vi "Wrapper_Get Image Frame.vi"(7 "Image Ref in":T4, 8 "error in (no error)":errorcluster, 9 "frameindex in":i32, 10 "LIMPICTURE in":T2, 11 "hFile in":T3) -> (0 "error out":errorcluster, 1 "LIMLOCALMETADATA":T1 {"dTimeMSec" format="%.2f"}, 2 "LIMPICTURE out":T2, 3 "hFile out":T3, 5 "Image Ref out":T4)   [LabVIEW 2014, in "ND2_Reader_32.lvlib"]
uses:
  ND2_Reader_32.lvlib
  <vilib>/vision/Image Controls.llb/IMAQ Image.ctl
  controls/numeric_LIMFILEHANDLE.ctl
  controls/cluster_LIMPICTURE.ctl
  controls/cluster_LIMLOCALMETADATA.ctl
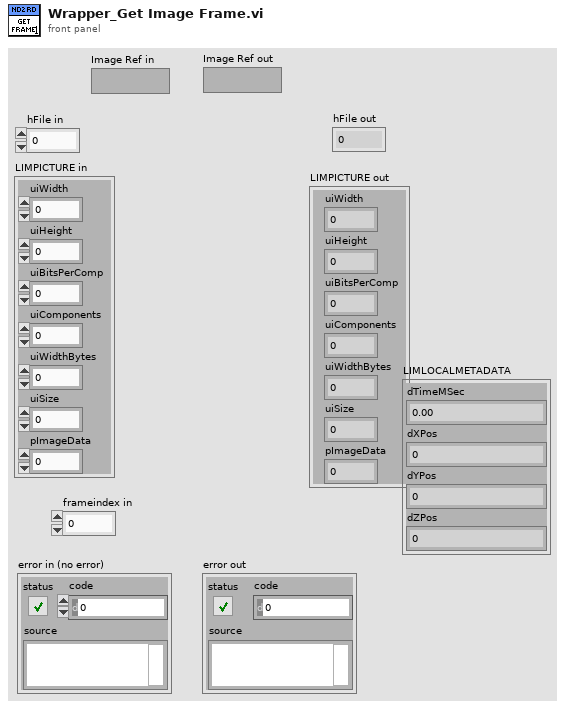
[diagram p1: front panel]
types:
  T1 = typedef "cluster_LIMLOCALMETADATA.ctl" = cluster{"dTimeMSec":dbl, "dXPos":dbl, "dYPos":dbl, "dZPos":dbl}
  T2 = typedef "cluster_LIMPICTURE.ctl" = cluster{"uiWidth":u32, "uiHeight":u32, "uiBitsPerComp":u32, "uiComponents":u32, "uiWidthBytes":u32, "uiSize":u32, "pImageData":u32}
  T3 = typedef "numeric_LIMFILEHANDLE.ctl" = i32
  T4 = typedef "IMAQ Image.ctl" = refnum<image>
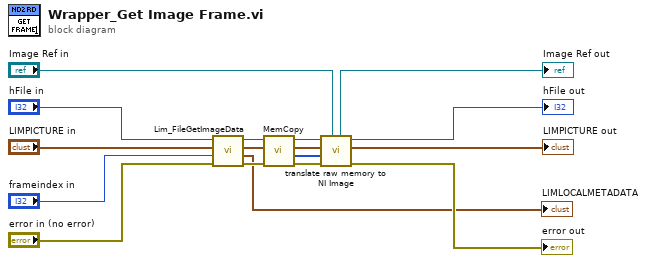
[diagram p0: block diagram]
diagram:
  n1 = call "Lim_FileGetImageData.vi"("error in (no error)"="error in (no error)", "frameindex"="frameindex in", "LIMPICTURE in"="LIMPICTURE in", "hFile in"="hFile in") -> ("error out"=w10:errorcluster, "LIMLOCALMETADATA"=→"LIMLOCALMETADATA":T1, "LIMPICTURE out"=w17:T2, "hFile out"=w11:T3)  [unwired: 4 in]
  n2 = call "MemCopy.vi"("error in (no error)"=w10, "LIMPICTURE in"=w17, "hFile in"=w11) -> ("error out"=w12:errorcluster, "pBuffer out"=w16:u8[], "LIMPICTURE out"=w15:T2, "hFile out"=w13:T3)  [unwired: 5 in]
  n3 = call "translate raw memory to NI Image.vi"("Image in"="Image Ref in", "error in (no error)"=w12, "pBuffer"=w16, "LIMPICTURE in"=w15, "hFile in"=w13) -> ("error out"=→"error out":errorcluster, "LIMPICTURE out"=→"LIMPICTURE out":T2, "hFile out"=→"hFile out":T3, "Image out"=→"Image Ref out":T4)  [unwired: 3 in]
